vi "Scan Add Write.vi"(7 "Write Value (0)":dbl, 8 "error in (no error)":errorcluster, 9 "Channel List(\"\")":string, 11 "VISA resource name":refnum<visa-resource-name>) -> (0 "error out":errorcluster, 3 "VISA resource name out":refnum<visa-resource-name>)   [LabVIEW 2015, in "Keithley DMM6500 DAQ6500 Series.lvlib"]
doc: "Adds channels to the scan list."
uses:
  <instrlib>/Keithley DMM6500 DAQ6500 Series/Keithley DMM6500 DAQ6500 Series.lvlib
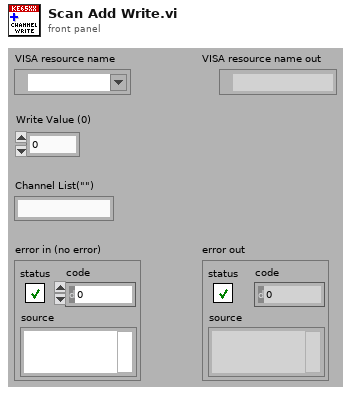
[diagram p1: front panel]
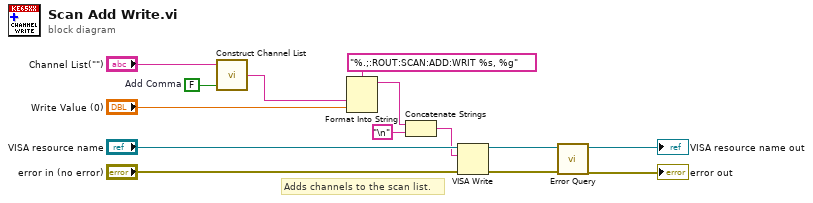
[diagram p0: block diagram]
diagram:
  w1 = FALSE  # Add Comma
  # "Adds channels to the scan list."
  n1 = call <instrlib>:"Construct Channel List.vi"("Add Comma (True)"=w1, "Channel List"="Channel List(\"\")") -> ("Channel List String"=w3:string)  [unwired: 1 in]
  n2 = Format Into String(format string="%.;:ROUT:SCAN:ADD:WRIT %s, %g", w3, "Write Value (0)") -> (resulting string=w5:string)  [unwired: 2 in, 1 out]
  n3 = Concatenate Strings(w5, "\n") -> (w6:string)
  n4 = VISA Write(VISA resource name="VISA resource name", write buffer=w6, error in (no error)="error in (no error)") -> (VISA resource name out=w10:refnum<visa-resource-name>, error out=w9:errorcluster)  [unwired: 1 out]
  n5 = call <instrlib>:"Error Query.vi"("error in (no error)"=w9, "VISA resource name"=w10) -> ("error out"=→"error out":errorcluster, "VISA resource name out"=→"VISA resource name out":refnum<visa-resource-name>)  [unwired: 6 in, 2 out]
